vi "AOTF_NonLinearLinesOnOff.vi"() -> ()   [LabVIEW 2013]
panel:
  in  "LineOnOff":bool[](array[boolean])
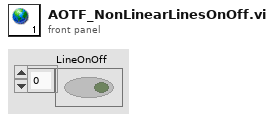
[diagram p1: front panel]
diagram:
